vi "BRig_dataTrial_I_anySelect_R.vi"() -> (2 "output_I_anySelect_R":i32)   [LabVIEW 2014]
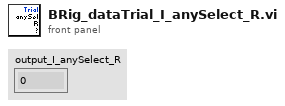
[diagram p1: front panel]
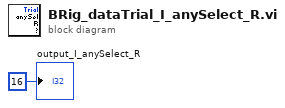
[diagram p0: block diagram]
diagram:
  "output_I_anySelect_R" <- 16 ("output_iBlock")
